vi "Init.vi"(6 "Event Self":map{string, refnum<data-value>}(c390), 8 "Queue Nested":map{string, refnum<data-value>}(c390), 9 "Queue Self":map{string, refnum<data-value>}(c390), 10 "Queue Caller":map{string, refnum<data-value>}(c390)) -> (3 "Base Event jettl out":refnum<class "Base Event jettl.lvclass">)   [LabVIEW 2021, in "jettl.lvlib" / "Base Event jettl.lvlib" / "Base Event jettl.lvclass"]
uses:
  Base Event jettl.lvclass
  Msg Strategy/Msg Strategy.lvclass
  State/Nominal State/Nominal State.lvclass
  C:/git/jettl/src/jettl/jettl/Base Event jettl/State/State/State.lvclass
  Base Event jettl.lvclass/Base Event jettl.ctl
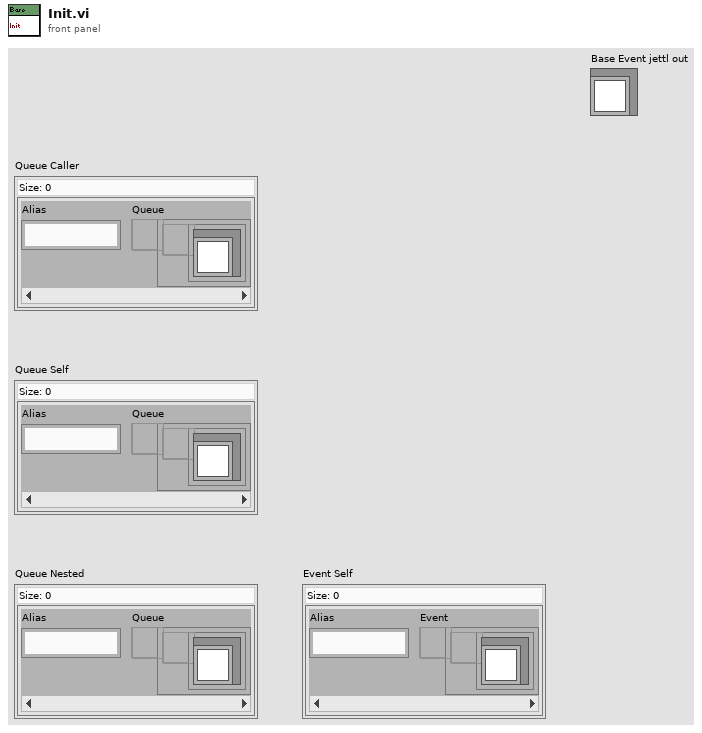
[diagram p1: front panel]
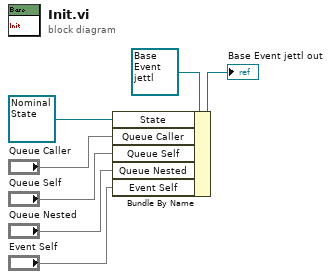
[diagram p0: block diagram]
diagram:
  n1 = Bundle By Name(cluster=refnum<class "Base Event jettl.lvclass"> refnum ("jettl Event Actor out"), "State"=refnum<class "Nominal State.lvclass"> refnum ("jettl.lvlib:Nominal Event State.lvclass"), "Queue Caller"="Queue Caller", "Queue Self"="Queue Self", "Queue Nested"="Queue Nested", "Event Self"="Event Self") -> (→"Base Event jettl out":refnum<class "Base Event jettl.lvclass">)
